vi "datatable.vi"(11 "Data Interface in":T1) -> (2 "Value String":string, 3 "Boolean":bool)   [LabVIEW 2013, in "data bus values.lvlib"]
uses:
  table/data bus values.lvlib
  table/data table.ctl
  tag/data bus tag description.lvclass
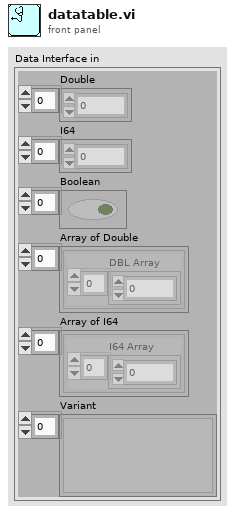
[diagram p1: front panel]
types:
  T1 = typedef "data bus values.lvlib/data table.ctl" = cluster{"Double":dbl[], "I64":i64[], "Boolean":bool[], "Array of Double":cluster{"DBL Array":dbl[]}[], "Array of I64":cluster{"I64 Array":i64[]}[], "Variant":variant[]}
  T2 = typedef "data bus tag description.lvclass/Data Type.ctl" = enum16{"Double", "I64", "Boolean", "Array of Double", "Array of I64", "Variant"}
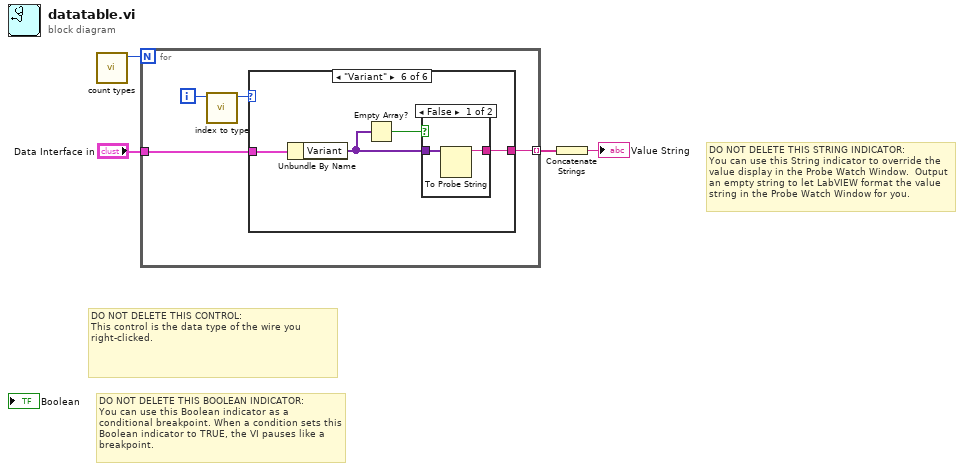
[diagram p0: block diagram]
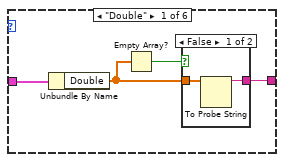
[diagram p2: hidden frame]
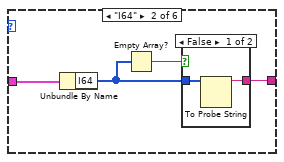
[diagram p4: hidden frame]
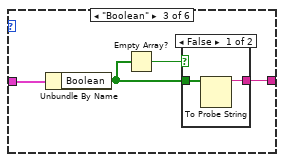
[diagram p6: hidden frame]
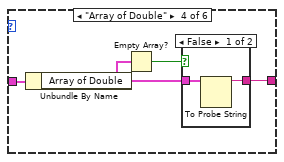
[diagram p8: hidden frame]
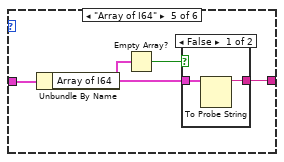
[diagram p10: hidden frame]
diagram:
  # "DO NOT DELETE THIS STRING INDICATOR: \nYou can use this String indicator to override the value display in the Probe Watch Window.  Output an empty string to let LabVIEW format the value string in the Probe Watch Window for you."
  # "DO NOT DELETE THIS BOOLEAN INDICATOR: \nYou can use this Boolean indicator as a conditional breakpoint. When a condition sets this Boolean indicator to TRUE, the VI pauses like a breakpoint."
  # "DO NOT DELETE THIS CONTROL: \nThis control is the data type of the wire you right-clicked."
  n1 = call "count types.vi"() -> ("type count"=w4:i32)  [unwired: 11 in]
  n2 = for {
    N: w4 -> [_]
    tunnel: "Data Interface in" -> [w7]
    tunnel: [w5] -> w2 mode=indexing
    i -> [w8]
    n3 = call "index to type.vi"("I32"=w8) -> ("type"=w6:T2)  [unwired: 10 in]
    n4 = case shown="\"Variant\"" w6 {
      tunnel: w7 -> [w12 w18 w24 w30 w36 w42]
      tunnel: [w9 w15 w21 w27 w33 w39] -> w5
      frame "Double" {
        n5 = Unbundle By Name(w12) -> ("Double"=w10:dbl[])
        n6 = Empty Array?(array=w10) -> (empty?=w11:bool)
        n7 = case shown="False" w11 {
          tunnel: w10 -> [w14 _]
          tunnel: [w13 _] -> w9
          frame False {
            n8 = To Probe String(7:w14) -> (3:w13:string)  [unwired: 2 in, 1 out]
          }
          frame True {
          }
        }
      }
      frame "I64" {
        n9 = Unbundle By Name(w18) -> ("I64"=w16:i64[])
        n10 = Empty Array?(array=w16) -> (empty?=w17:bool)
        n11 = case shown="False" w17 {
          tunnel: w16 -> [w20 _]
          tunnel: [w19 _] -> w15
          frame False {
            n12 = To Probe String(7:w20) -> (3:w19:string)  [unwired: 2 in, 1 out]
          }
          frame True {
          }
        }
      }
      frame "Boolean" {
        n13 = Unbundle By Name(w24) -> ("Boolean"=w22:bool[])
        n14 = Empty Array?(array=w22) -> (empty?=w23:bool)
        n15 = case shown="False" w23 {
          tunnel: w22 -> [w26 _]
          tunnel: [w25 _] -> w21
          frame False {
            n16 = To Probe String(7:w26) -> (3:w25:string)  [unwired: 2 in, 1 out]
          }
          frame True {
          }
        }
      }
      frame "Array of Double" {
        n17 = Unbundle By Name(w30) -> ("Array of Double"=w28:cluster{"DBL Array":dbl[]}[])
        n18 = Empty Array?(array=w28) -> (empty?=w29:bool)
        n19 = case shown="False" w29 {
          tunnel: w28 -> [w32 _]
          tunnel: [w31 _] -> w27
          frame False {
            n20 = To Probe String(7:w32) -> (3:w31:string)  [unwired: 2 in, 1 out]
          }
          frame True {
          }
        }
      }
      frame "Array of I64" {
        n21 = Unbundle By Name(w36) -> ("Array of I64"=w34:cluster{"I64 Array":i64[]}[])
        n22 = Empty Array?(array=w34) -> (empty?=w35:bool)
        n23 = case shown="False" w35 {
          tunnel: w34 -> [w38 _]
          tunnel: [w37 _] -> w33
          frame False {
            n24 = To Probe String(7:w38) -> (3:w37:string)  [unwired: 2 in, 1 out]
          }
          frame True {
          }
        }
      }
      frame "Variant" {
        n25 = Unbundle By Name(w42) -> ("Variant"=w40:variant[])
        n26 = Empty Array?(array=w40) -> (empty?=w41:bool)
        n27 = case shown="False" w41 {
          tunnel: w40 -> [w44 _]
          tunnel: [w43 _] -> w39
          frame False {
            n28 = To Probe String(7:w44) -> (3:w43:string)  [unwired: 2 in, 1 out]
          }
          frame True {
          }
        }
      }
    }
  }
  n29 = Concatenate Strings(w2) -> (→"Value String":string)
